vi "Destroy Subscription.vi"(8 "error in (no error)":errorcluster, 11 "Subscription in":refnum<class "Subscription.lvclass">) -> (0 "error out":errorcluster, 3 "Subscription out":refnum<class "Subscription.lvclass">)   [LabVIEW 2013, in "MQTT Base.lvlib" / "Subscription.lvclass"]
uses:
  Subscription.lvclass
  Subscription.lvclass/Subscription.ctl
  TopicFilter/TopicFilter.lvclass
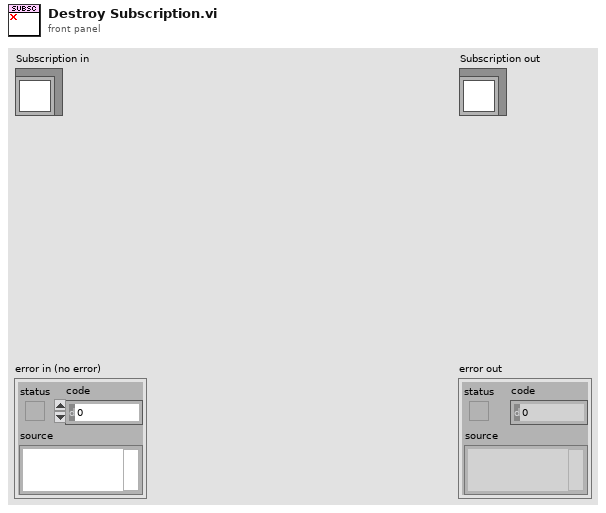
[diagram p1: front panel]
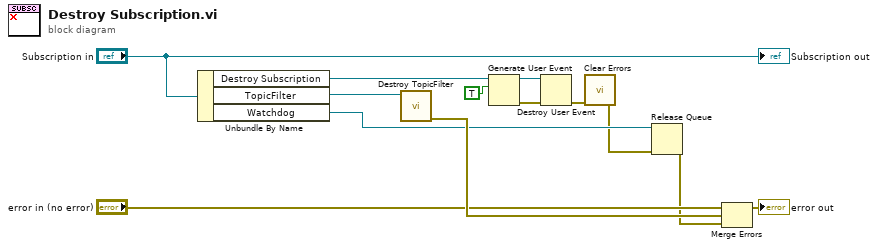
[diagram p0: block diagram]
diagram:
  n1 = Unbundle By Name("Subscription in") -> ("Destroy Subscription"=w8:refnum<user-event>, "TopicFilter"=w12:refnum<class "TopicFilter.lvclass">, "Watchdog"=w3:refnum<queue>)
  n2 = call "Destroy TopicFilter.vi"("TopicFilter in"=w12) -> ("error out"=w11:errorcluster)  [unwired: 9 in, 1 out]
  n3 = Generate User Event(user event=w8, event data cluster=TRUE ("event data")) -> (user event out=w6:refnum<user-event>, error out=w5:errorcluster)  [unwired: 2 in]
  n4 = Destroy User Event(user event=w6, error in=w5) -> (error out=w4:errorcluster)
  n5 = call <vilib>:"Clear Errors.vi"("error in (no error)"=w4) -> ("error out"=w2:errorcluster)  [unwired: 6 in]
  n6 = Release Queue(queue=w3, error in (no error)=w2) -> (error out=w1:errorcluster)  [unwired: 1 in, 2 out]
  n7 = Merge Errors("error in (no error)", w11, w1) -> (→"error out":errorcluster)
  "Subscription out" <- "Subscription in"
